vi "获取优势程度数组.vi"(1 "输入数组":T1(array[cluster])) -> (0 "输出数组":dbl[](array[numeric]))   [LabVIEW 2017]
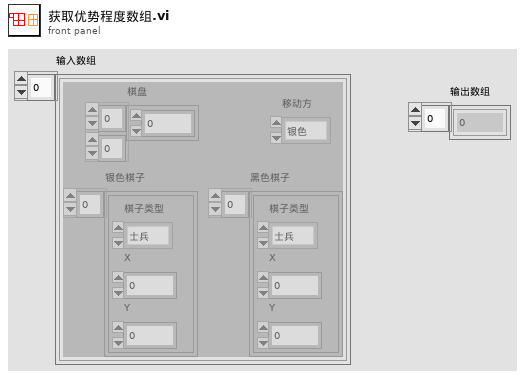
[diagram p1: front panel]
types:
  T1 = cluster{"棋盘":u16[][], "银色棋子":cluster{"棋子类型":enum16{"士兵", "骑士", "主教", "战车", "皇后", "国王", "空"}, "X":u8, "Y":u8}[], "黑色棋子":cluster{"棋子类型":enum16{"士兵", "骑士", "主教", "战车", "皇后", "国王", "空"}, "X":u8, "Y":u8}[], "移动方":enum16{"银色", "黑色"}}[]
  T2 = cluster{"棋盘":u16[][], "银色棋子":cluster{"棋子类型":enum16{"士兵", "骑士", "主教", "战车", "皇后", "国王", "空"}, "X":u8, "Y":u8}[], "黑色棋子":cluster{"棋子类型":enum16{"士兵", "骑士", "主教", "战车", "皇后", "国王", "空"}, "X":u8, "Y":u8}[], "移动方":enum16{"银色", "黑色"}}
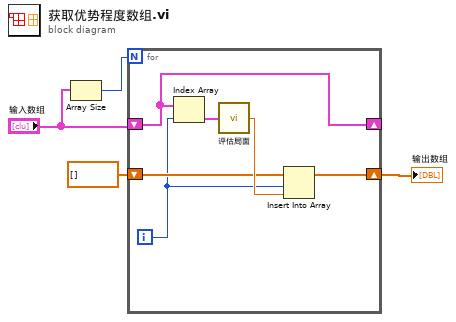
[diagram p0: block diagram]
diagram:
  n1 = Array Size(array="输入数组") -> (size(s)=w3:i32)
  n2 = for {
    N: w3 -> [_]
    shift-right: [w9] -> _
    shift-left: "输入数组" -> [w9]
    shift-right: [w6] -> w1
    shift-left: dbl[] [] -> [w7]
    i -> [w5]
    n3 = Index Array(array=w9, index=w5) -> (element=w10:T2)
    n4 = call "评估局面.vi"("输入的棋盘"=w10) -> ("优势程度"=w8:dbl)
    n5 = Insert Into Array(array=w7, index=w5, new element=w8) -> (w6:dbl[])
  }
  "输出数组" <- w1
